vi "logic-train-sample-7-1.vi"(11 "Request\nCapture":bool) -> (1 "Hand_Close":bool, 3 "Arm_Extend":bool, 4 "State":T1)   [LabVIEW 2020]
uses:
  sample-7-1-state-enum.ctl
  <vilib>/Utility/semaphor.llb/Obtain Semaphore Reference.vi
  <vilib>/Rock Robotics/WPI/ThirdParty/JAS_Junk/TrajLib/Timer_Reset.vi
  <vilib>/Rock Robotics/WPI/ThirdParty/JAS_Junk/TrajLib/Timer_Start.vi
  <vilib>/Rock Robotics/WPI/ThirdParty/JAS_Junk/TrajLib/Timer_Stop.vi
  <vilib>/Rock Robotics/WPI/ThirdParty/JAS_Junk/TrajLib/Trajectory_Library.lvlib
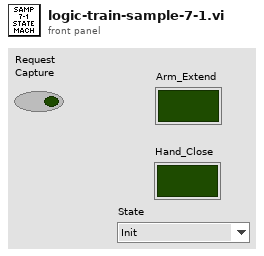
[diagram p1: front panel]
types:
  T1 = typedef "sample-7-1-state-enum.ctl" = enum16{"Init", "ExtendArm", "ExtendArmWait", "CloseHand", "CloseHandWait", "RetractArm", "RetractArmWait", "OpenHand", "OpenHandWait", "Ready"}
  T2 = typedef "Trajectory_Library.lvlib/TIMER.ctl" = cluster{"StartTime":dbl, "Accumulated TIme":dbl, "Running":bool, "semaphore":T3}
  T3 = typedef "Semaphore RefNum" = refnum<k1>
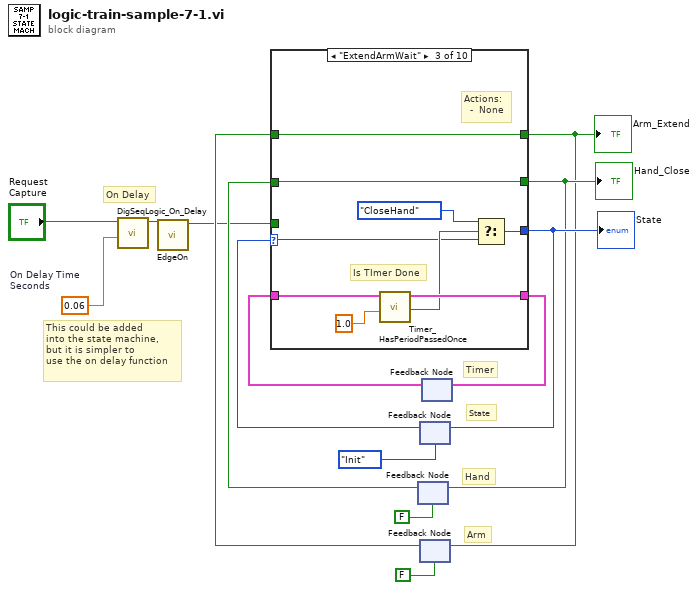
[diagram p0: block diagram]
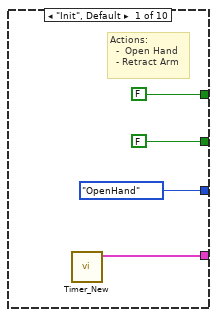
[diagram p2: hidden frame]
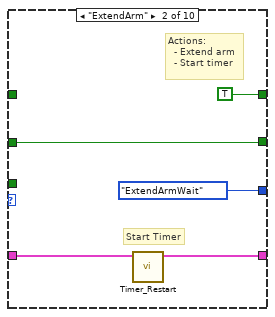
[diagram p3: hidden frame]
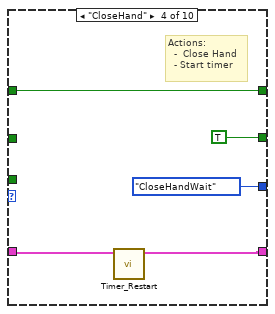
[diagram p4: hidden frame]
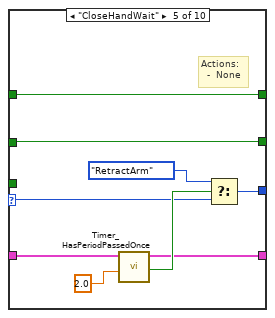
[diagram p5: hidden frame]
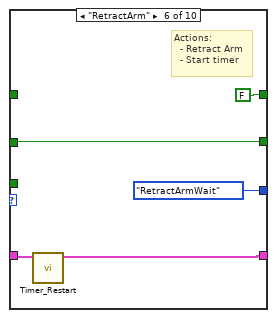
[diagram p6: hidden frame]
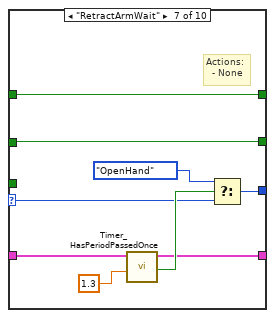
[diagram p7: hidden frame]
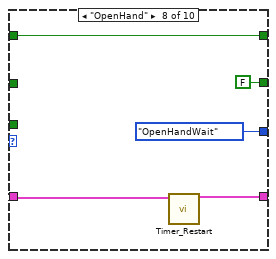
[diagram p8: hidden frame]
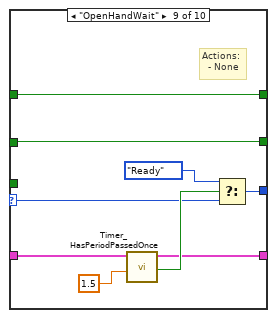
[diagram p9: hidden frame]
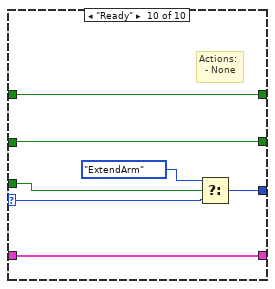
[diagram p10: hidden frame]
diagram:
  w4 = 0.06  # On Delay Time Seconds
  # "This could be added\ninto the state machine,\nbut it is simpler to \nuse the on delay function"
  # "On Delay"
  # "State"
  # "Timer"
  # "Arm"
  # "Hand"
  n1 = call <vilib>:"DigSeqLogic_On_Delay.vi"("Delay"=w4, "Input"="Request\nCapture") -> ("Output"=w3:bool)  [unwired: 8 in, 1 out]
  n2 = call "EdgeOn.vi"("Input"=w3) -> ("Edge On"=w1:bool)  [unwired: 10 in]
  n3 = feedback #1(FALSE) -> (w6:bool)
  n4 = feedback #2(sample-7-1-state-enum."Init" ("Sample-7-1-State")) -> (w14:T1)
  n5 = feedback #3(FALSE) -> (w5:bool)
  n6 = feedback #4() -> (w7:T2)  [unwired: 1 in]
  n7 = case shown="\"ExtendArmWait\"" w14 {
    selector: w14 -> [_ _ w25 _ w43 _ w58 _ w71 w78]
    tunnel: [FALSE TRUE w32 w38 w39 FALSE w54 w63 w67 w82] -> w11
    tunnel: [FALSE w23 w33 TRUE w40 w49 w53 FALSE w68 w81] -> w12
    tunnel: [sample-7-1-state-enum."OpenHand" ("Sample-7-1-State") sample-7-1-state-enum."ExtendArmWait" ("Sample-7-1-State") w27 sample-7-1-state-enum."CloseHandWait" ("Sample-7-1-State") w44 sample-7-1-state-enum."RetractArmWait" ("Sample-7-1-State") w57 sample-7-1-state-enum."OpenHandWait" ("Sample-7-1-State") w72 w76] -> w13
    tunnel: [w16 w20 w30 w37 w41 w52 w55 w65 w69 w80] -> w8
    tunnel: w7 -> [_ w21 w29 w36 w42 w48 w56 w64 w70 w80]
    tunnel: w6 -> [_ w23 w33 _ w40 w49 w53 _ w68 w81]
    tunnel: w5 -> [_ _ w32 w38 w39 _ w54 w63 w67 w82]
    tunnel: w1 -> [_ _ _ _ _ _ _ _ _ w79]
    frame "Init", Default {
      # "Actions:\n  -  Open Hand\n  - Retract Arm"
      n8 = call <vilib>:"Timer_New.vi"() -> ("TIMER"=w16:T2)  [unwired: 11 in]
    }
    frame "ExtendArm" {
      # "Start Timer"
      # "Actions:\n  - Extend arm\n  - Start timer"
      n9 = call <vilib>:"Timer_Restart.vi"("in Timer"=w21) -> ("out Timer"=w20:T2)  [unwired: 10 in]
    }
    frame "ExtendArmWait" {
      # "Is TImer Done"
      # "Actions:\n  -  None"
      n10 = call <vilib>:"Timer_HasPeriodPassedOnce.vi"("Period"=1.0, "in Timer"=w29) -> ("Expired"=w26:bool, "out Timer"=w30:T2)  [unwired: 7 in, 1 out]
      n11 = Select(t=sample-7-1-state-enum."CloseHand" ("Sample-7-1-State"), s=w26, f=w25) -> (s? t:f=w27:T1)
    }
    frame "CloseHand" {
      # "Actions:\n  -  Close Hand\n  - Start timer"
      n12 = call <vilib>:"Timer_Restart.vi"("in Timer"=w36) -> ("out Timer"=w37:T2)  [unwired: 10 in]
    }
    frame "CloseHandWait" {
      # "Actions:\n  -  None"
      n13 = call <vilib>:"Timer_HasPeriodPassedOnce.vi"("Period"=2.0, "in Timer"=w42) -> ("Expired"=w45:bool, "out Timer"=w41:T2)  [unwired: 7 in, 1 out]
      n14 = Select(t=sample-7-1-state-enum."RetractArm" ("Sample-7-1-State"), s=w45, f=w43) -> (s? t:f=w44:T1)
    }
    frame "RetractArm" {
      # "Actions:\n  - Retract Arm\n  - Start timer"
      n15 = call <vilib>:"Timer_Restart.vi"("in Timer"=w48) -> ("out Timer"=w52:T2)  [unwired: 10 in]
    }
    frame "RetractArmWait" {
      # "Actions:\n  - None"
      n16 = call <vilib>:"Timer_HasPeriodPassedOnce.vi"("Period"=1.3, "in Timer"=w56) -> ("Expired"=w59:bool, "out Timer"=w55:T2)  [unwired: 7 in, 1 out]
      n17 = Select(t=sample-7-1-state-enum."OpenHand" ("Sample-7-1-State"), s=w59, f=w58) -> (s? t:f=w57:T1)
    }
    frame "OpenHand" {
      n18 = call <vilib>:"Timer_Restart.vi"("in Timer"=w64) -> ("out Timer"=w65:T2)  [unwired: 10 in]
    }
    frame "OpenHandWait" {
      # "Actions:\n  - None"
      n19 = call <vilib>:"Timer_HasPeriodPassedOnce.vi"("Period"=1.5, "in Timer"=w70) -> ("Expired"=w73:bool, "out Timer"=w69:T2)  [unwired: 7 in, 1 out]
      n20 = Select(t=sample-7-1-state-enum."Ready" ("Sample-7-1-State"), s=w73, f=w71) -> (s? t:f=w72:T1)
    }
    frame "Ready" {
      # "Actions:\n  - None"
      n21 = Select(t=sample-7-1-state-enum."ExtendArm", s=w79, f=w78) -> (s? t:f=w76:T1)
    }
  }
  "State" <- w13
  "Arm_Extend" <- w11
  "Hand_Close" <- w12
  n22 = feedback-in #1(w12) -> ()
  n23 = feedback-in #2(w13) -> ()
  n24 = feedback-in #3(w11) -> ()
  n25 = feedback-in #4(w8) -> ()
